vi "InitializeAcquisitionSession.vi"(8 "error in (no error)":errorcluster, 11 "Photometrics_CH-250_CamIn":refnum<class "Photometrics_CH-250_Cam.lvclass">) -> (0 "error out":errorcluster, 3 "Photometrics Cam v2 out":refnum<class "Photometrics_CH-250_Cam.lvclass">)   [LabVIEW 2013, in "Photometrics_CH-250_Cam.lvclass"]
doc: "This VI (1) initializes the camera communication, (2) creates and IMAQimage, (3) sets the ADCoffsetparameter and (4) sets the camera (trigger, exposure, region)"
uses:
  Photometrics_CH-250_Cam.lvclass
  SubVis/DLL Calls/PARAM_ID_TypDef.ctl
  CameraSessionClass/CS250-CameraHardwareClass.lvclass
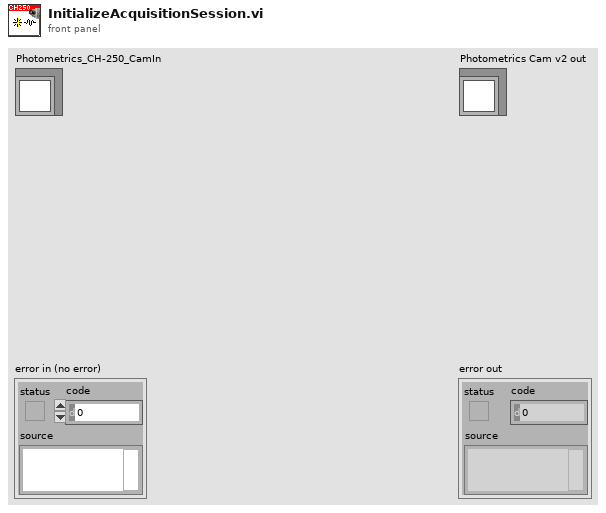
[diagram p1: front panel]
types:
  T1 = typedef "PARAM_ID_TypDef.ctl" = u32
  T2 = typedef "OnOffTypeDef.ctl" = enum16{"off", "on"}
  T3 = typedef "TriggerMode_TypDef.ctl" = enum16{"Timed", "Strobed", "Bulb", "Trigger first", "Flash", "Variable Timed"}
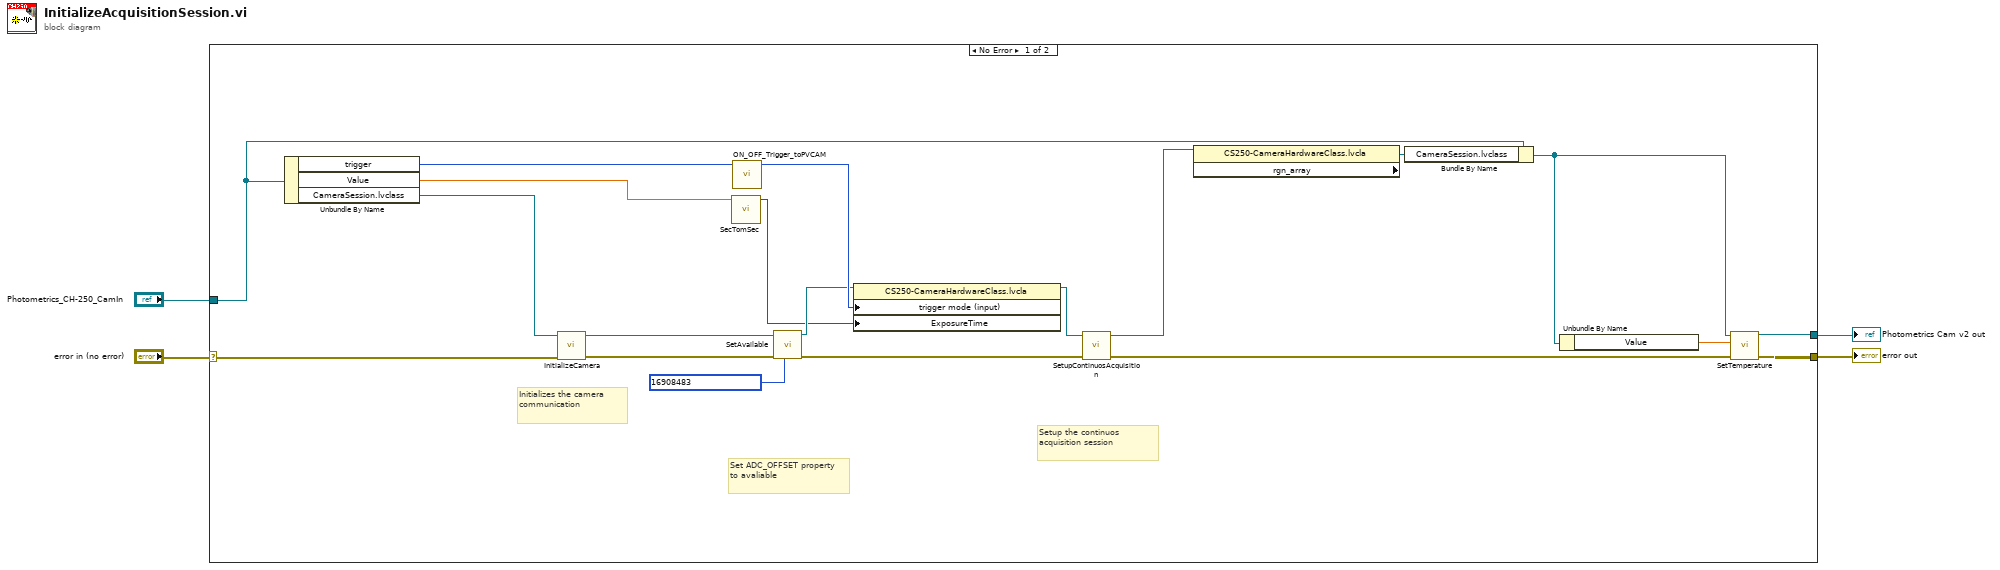
[diagram p0: block diagram]
diagram:
  n1 = case shown="No Error" "error in (no error)" {
    selector: "error in (no error)" -> [w16 w26]
    tunnel: [w7 w26] -> w3
    tunnel: [w6 w25] -> w1
    tunnel: "Photometrics_CH-250_CamIn" -> [w12 w25]
    frame No Error {
      # "Setup the continuos acquisition session"
      # "Set ADC_OFFSET property to avaliable"
      # "Initializes the camera communication"
      n2 = Unbundle By Name(w12) -> ("trigger"=w24:T2, "Value"=w23:dbl, "CameraSession.lvclass"=w13:refnum<class "CS250-CameraHardwareClass.lvclass">)
      n3 = call-dynamic "InitializeCamera.vi"("error in (no error)"=w16, "CameraSession in"=w13) -> ("error out"=w11:errorcluster, "CameraSession out"=w10:refnum<class "CS250-CameraHardwareClass.lvclass">)  [unwired: 8 in]
      n4 = call "SecTomSec.vi"("Sec"=w23) -> ("mSec"=w5:u32)  [unwired: 10 in]
      n5 = call "ON_OFF_Trigger_toPVCAM.vi"("Trigger"=w24) -> ("trigger mode (input)"=w22:T3)  [unwired: 10 in]
      n6 = call-dynamic "SetAvailable.vi"("Param ID (Ring)"=T1 16908483, "error in (no error)"=w11, "CameraSession in"=w10) -> ("error out"=w20:errorcluster, "CameraSession out"=w19:refnum<class "CS250-CameraHardwareClass.lvclass">)  [unwired: 7 in]
      n7 = property class="CS250-CameraHardwareClass.lvcla"(reference=w19, "trigger mode (input)"=w22, "ExposureTime"=w5) -> (reference out=w21:refnum<class "CS250-CameraHardwareClass.lvclass">)  [unwired: 1 in, 1 out]
      n8 = call-dynamic "SetupContinuosAcquisition.vi"("error in (no error)"=w20, "CameraSession in"=w21) -> ("error out"=w8:errorcluster, "CameraSession out"=w9:refnum<class "CS250-CameraHardwareClass.lvclass">)  [unwired: 8 in]
      n9 = property class="CS250-CameraHardwareClass.lvcla" props=["rgn_array"](reference=w9) -> (reference out=w17:refnum<class "CS250-CameraHardwareClass.lvclass">)  [unwired: 1 in, 2 out]
      n10 = Bundle By Name(cluster=w12, "CameraSession.lvclass"=w17) -> (w14:refnum<class "Photometrics_CH-250_Cam.lvclass">)
      n11 = Unbundle By Name(w14) -> ("Value"=w15:dbl)
      n12 = call-dynamic "SetTemperature.vi"("error in (no error)"=w8, "Temperature(degC)"=w15, "Photometrics Cam v2 in"=w14) -> ("error out"=w7:errorcluster, "Photometrics Cam v2 out"=w6:refnum<class "Photometrics_CH-250_Cam.lvclass">)  [unwired: 6 in, 1 out]
    }
    frame Error {
    }
  }
  "error out" <- w3
  "Photometrics Cam v2 out" <- w1
